vi "MAIN.vi"() -> ()   [LabVIEW 2019]
uses:
  current_values_cluster_typedef.ctl
  states_enum_typedef.ctl
  <vilib>/Instr/_visa.llb/VISA Configure Serial Port (Instr).vi
panel:
  out "Current Values":T1
  out "Error Out":errorcluster
  in  "Connect":bool
  in  "COM Port":refnum<visa-resource-name>
  out "Output Chart":dbl(graph)
  in  "Set":bool
  in  "Stop":bool
  in  "SP":dbl
  in  "Kd":dbl
  in  "Ki":dbl
  in  "Kp":dbl
  out "PV SP Chart":cluster{"SP":dbl, "PV":dbl}(graph)
  # "PID Controller"
  # "Instructions\n1) Select the COM port and click Connect\n2) Adjust gains and set points, click Set to make\n     changes active\n3) Observe output\n4) When done, click stop to disconnect and exit"
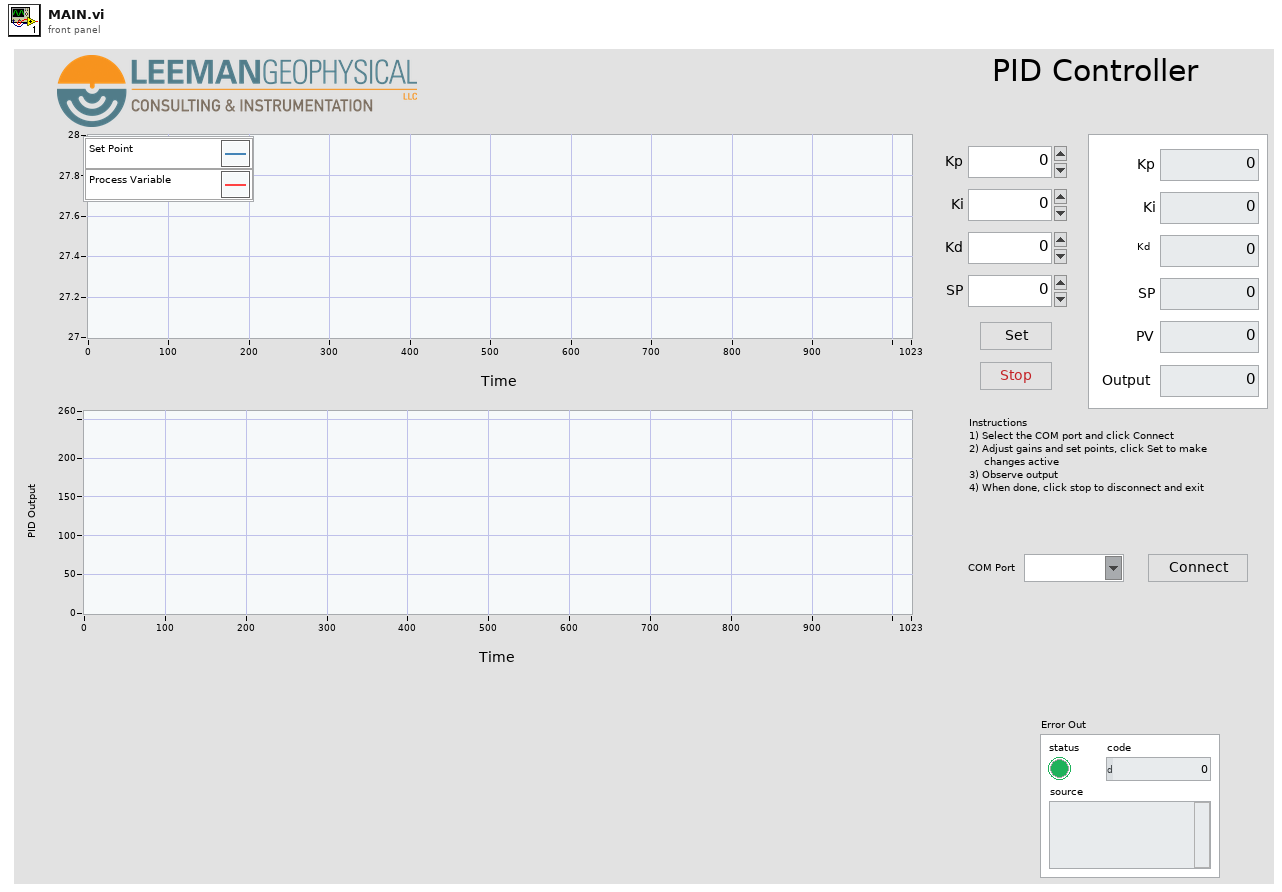
[diagram p1: front panel]
types:
  T1 = typedef "current_values_cluster_typedef.ctl" = cluster{"Kp":dbl, "Ki":dbl, "Kd":dbl, "SP":dbl, "PV":dbl, "Output":dbl}
  T2 = typedef "states_enum_typedef.ctl" = enum16{"Connect", "Poll", "Initialize", "Shutdown", "Read", "Set"}
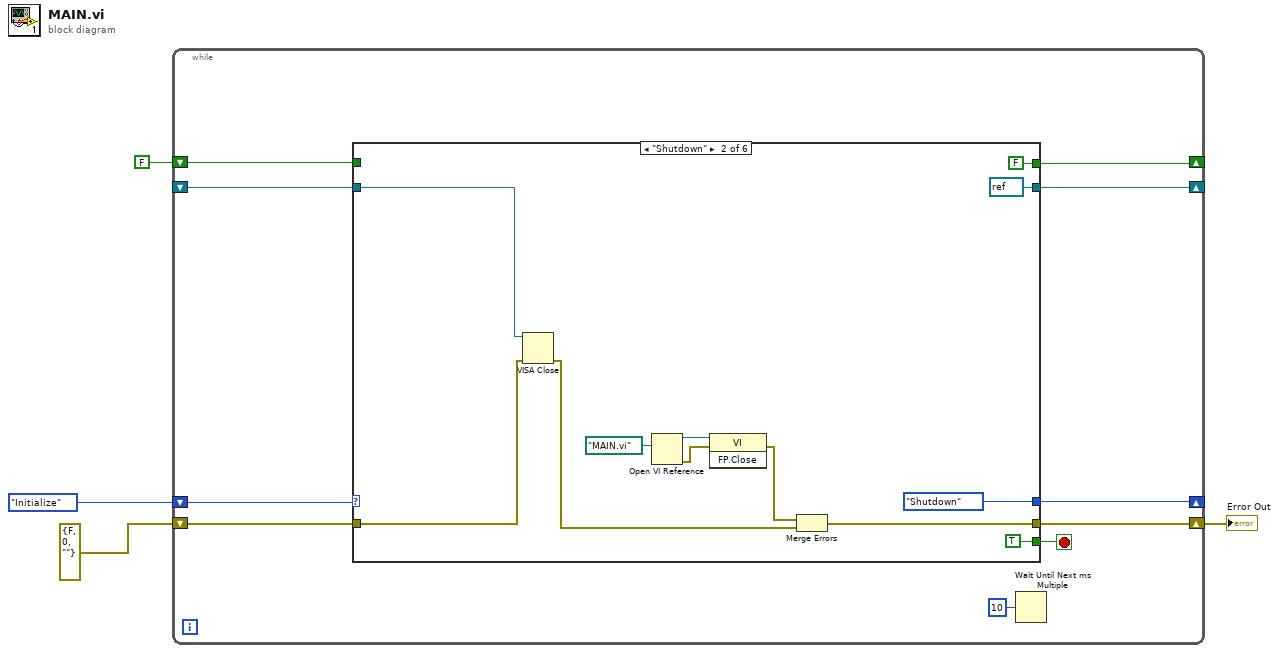
[diagram p0: block diagram]
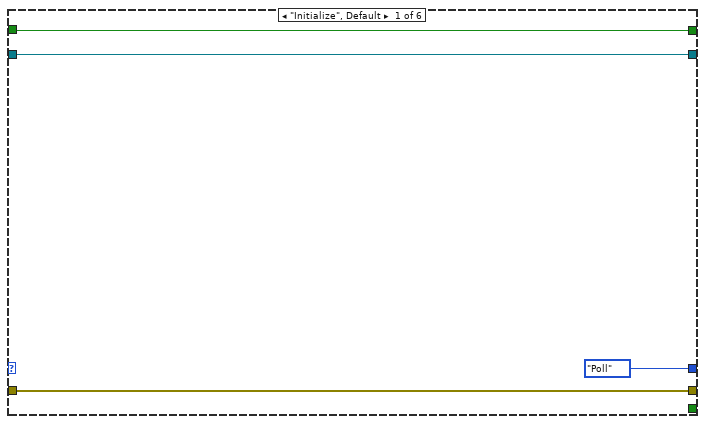
[diagram p2: hidden frame]
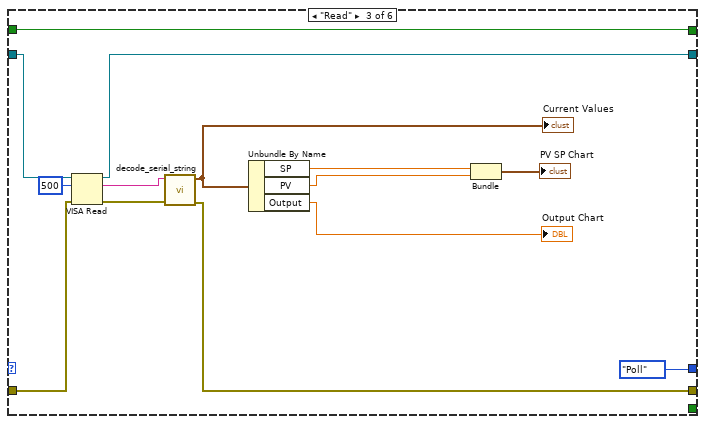
[diagram p3: hidden frame]
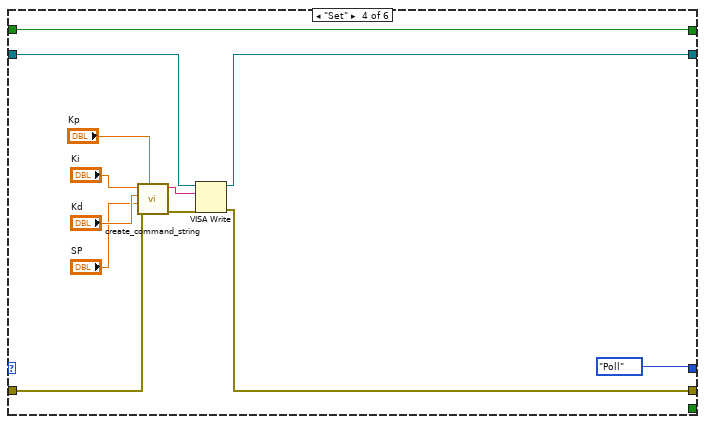
[diagram p4: hidden frame]
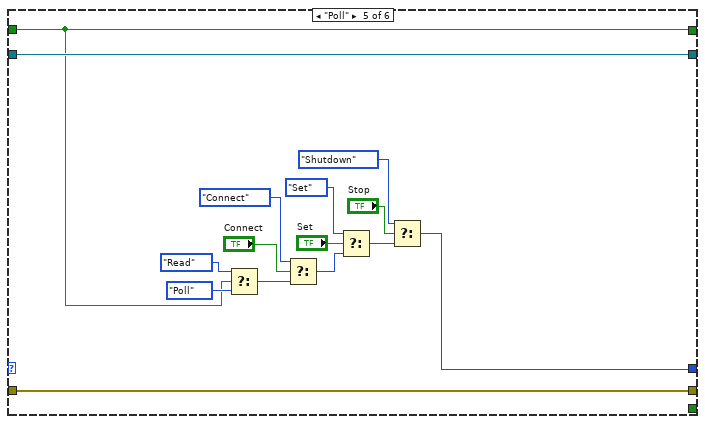
[diagram p5: hidden frame]
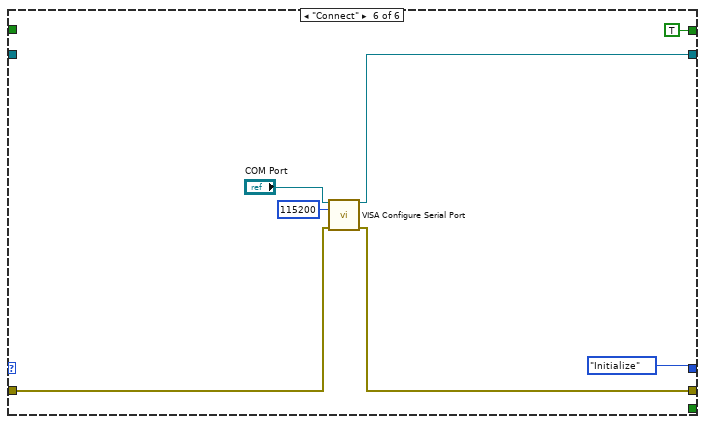
[diagram p6: hidden frame]
diagram:
  n1 = while {
    shift-right: [w13] -> _
    shift-left: states_enum_typedef."Initialize" -> [w14]
    shift-right: [w6] -> _
    shift-left: FALSE -> [w10]
    shift-right: [w8] -> w2
    shift-left: errorcluster {"status"=FALSE, "code"=0, "source"=""} ("error out") -> [w9]
    shift-right: [w7] -> _
    shift-left: _ -> [w5]
    stop <- w11 stop-if-true
    n2 = case shown="\"Shutdown\"" w14 {
      tunnel: [states_enum_typedef."Poll" states_enum_typedef."Shutdown" states_enum_typedef."Poll" states_enum_typedef."Poll" w66 states_enum_typedef."Initialize"] -> w13
      tunnel: [_ TRUE _ _ _ _] -> w11
      tunnel: w10 -> [w16 _ w40 w46 w57 _]
      tunnel: w9 -> [w17 w25 w42 w51 w58 w75]
      tunnel: [w17 w21 w37 w45 w58 w74] -> w8
      tunnel: [w15 refnum<visa-resource-name> refnum ("VISA resource name out") w41 w47 w59 w73] -> w7
      tunnel: [w16 FALSE w40 w46 w57 TRUE] -> w6
      tunnel: w5 -> [w15 w26 w43 w48 w59 _]
      frame "Initialize", Default {
      }
      frame "Shutdown" {
        n3 = VISA Close(VISA resource name=w26, error in (no error)=w25) -> (error out=w19:errorcluster)
        n4 = Open VI Reference(vi path=path "MAIN.vi") -> (vi reference=w23:refnum<vi>, error out=w24:errorcluster)  [unwired: 5 in]
        n5 = invoke class="VI" method="FP.Close"(reference=w23, error in=w24) -> (error out=w20:errorcluster)  [unwired: 1 in, 2 out]
        n6 = Merge Errors(w20, w19) -> (w21:errorcluster)
      }
      frame "Read" {
        n7 = VISA Read(VISA resource name=w43, byte count=u32 500, error in (no error)=w42) -> (VISA resource name out=w41:refnum<visa-resource-name>, read buffer=w38:string, error out=w39:errorcluster)  [unwired: 1 out]
        n8 = call "decode_serial_string.vi"("Error In"=w39, "Input Str"=w38) -> ("Error Out"=w37:errorcluster, "Current Values"=w35:T1)  [unwired: 7 in, 1 out]
        "Current Values" <- w35
        n9 = Unbundle By Name(w35) -> ("SP"=w34:dbl, "PV"=w33:dbl, "Output"=→"Output Chart":dbl)
        n10 = Bundle("SP"=w34, "PV"=w33) -> (→"PV SP Chart":cluster{"SP":dbl, "PV":dbl})  [unwired: 1 in]
      }
      frame "Set" {
        n11 = call "create_command_string.vi"("Kp"="Kp", "Error In"=w51, "SP"="SP", "Kd"="Kd", "Ki"="Ki") -> ("Error Out"=w50:errorcluster, "concatenated string"=w49:string)  [unwired: 5 in]
        n12 = VISA Write(VISA resource name=w48, write buffer=w49, error in (no error)=w50) -> (VISA resource name out=w47:refnum<visa-resource-name>, error out=w45:errorcluster)  [unwired: 1 out]
      }
      frame "Poll" {
        n13 = Select(t=states_enum_typedef."Read", s=w57, f=states_enum_typedef."Poll") -> (s? t:f=w63:T2)
        n14 = Select(t=states_enum_typedef."Connect", s="Connect", f=w63) -> (s? t:f=w60:T2)
        n15 = Select(t=states_enum_typedef."Set", s="Set", f=w60) -> (s? t:f=w67:T2)
        n16 = Select(t=states_enum_typedef."Shutdown", s="Stop", f=w67) -> (s? t:f=w66:T2)
      }
      frame "Connect" {
        n17 = call-poly "VISA Configure Serial Port"("VISA resource name"="COM Port", "baud rate (9600)"=u32 115200, "error in (no error)"=w75) -> ("VISA resource name out"=w73:refnum<visa-resource-name>, "error out"=w74:errorcluster)  [unwired: 11 in]
      }
    }
    n18 = Wait Until Next ms Multiple(millisecond multiple=u32 10) -> ()  [unwired: 1 out]
  }
  "Error Out" <- w2
